vi "DisableSingle.vi"(6 "return immediately":bool, 8 "error in (no error)":errorcluster, 10 "axis name":string, 11 "controller in":refnum<k24>) -> (0 "error out":errorcluster, 3 "controller out":refnum<k24>)   [LabVIEW 2020]
uses:
  C:/GEECS/Developers Version/source/Device Drivers/AerotechStage/Dlls/Aerotech.Ensemble.LabVIEW.dll
  Dlls/Aerotech.Ensemble.LabVIEW.dll
  C:/GEECS/Developers Version/source/Device Drivers/AerotechStage/Dlls/Aerotech.Ensemble.dll
  Dlls/Aerotech.Ensemble.dll
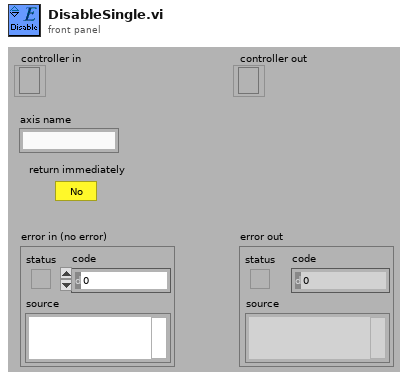
[diagram p1: front panel]
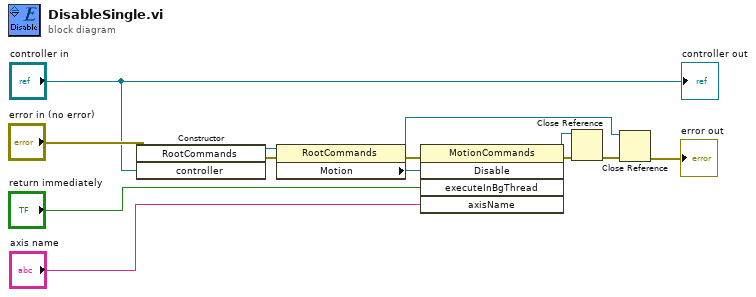
[diagram p0: block diagram]
diagram:
  n1 = constructor class="RootCommands"(error in="error in (no error)", "controller"="controller in") -> (reference out=w3:refnum<k24>, error out=w4:errorcluster)  [unwired: 2 in, 2 out]
  n2 = property class="RootCommands"(reference=w3, error in=w4) -> (reference out=w8:refnum<k24>, error out=w2:errorcluster, "Motion"=w1:refnum<k24>)
  n3 = invoke class="MotionCommands" method="Disable"(reference=w1, error in=w2, "executeInBgThread"="return immediately", "axisName"="axis name") -> (reference out=w6:refnum<k24>, error out=w5:errorcluster)  [unwired: 1 in, 3 out]
  n4 = Close Reference(reference=w6, error in (no error)=w5) -> (error out=w7:errorcluster)
  n5 = Close Reference(reference=w8, error in (no error)=w7) -> (error out=→"error out":errorcluster)
  "controller out" <- "controller in"
